vi "binarySearch.vi"(2 "Target":variant, 3 "Array":variant[](array[variant])) -> (0 "Itr to complete":i32, 1 "Result":i32)   [LabVIEW 2020]
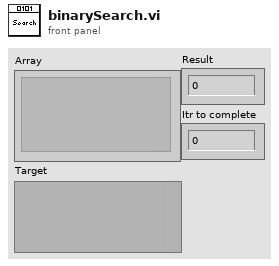
[diagram p1: front panel]
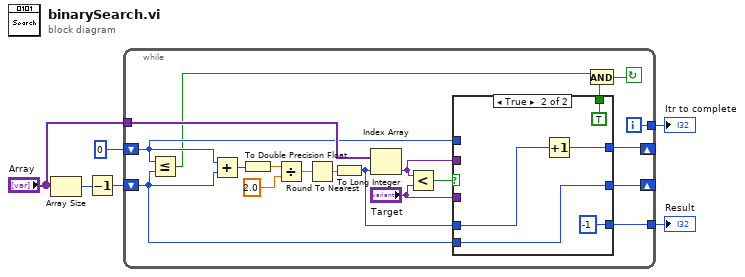
[diagram p0: block diagram]
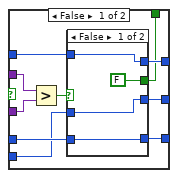
[diagram p2: hidden frame]
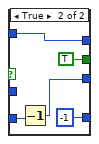
[diagram p3: hidden frame]
diagram:
  n1 = Array Size(array="Array") -> (size(s)=w6:i32)
  n2 = Decrement(x=w6) -> (x-1=w4:i32)
  n3 = while {
    tunnel: "Array" -> [w20]
    shift-right: [w18] -> _
    shift-left: 0 -> [w11]
    shift-right: [w14] -> _
    shift-left: w4 -> [w12]
    tunnel: [w13] -> w2
    tunnel: [w10] -> w1
    i -> [w10]
    stop <- w9 continue-if-true
    n4 = Less Or Equal?(x=w11, y=w12) -> (x <= y?=w8:bool)
    n5 = Add(x=w11, y=w12) -> (x+y=w25:i32)
    n6 = To Double Precision Float(number=w25) -> (double precision float=w24:dbl)
    n7 = Divide(x=w24, y=2.0) -> (x/y=w22:dbl)
    n8 = Round To Nearest(number=w22) -> (nearest integer value=w21:dbl)
    n9 = To Long Integer(number=w21) -> (32bit integer=w15:i32)
    n10 = Index Array(array=w20, index=w15) -> (element=w17:variant)
    n11 = Less?(x=w17, y="Target") -> (x < y?=w19:bool)
    n12 = case shown="True" w19 {
      tunnel: w15 -> [w32 w48]
      tunnel: [w28 w49] -> w18
      tunnel: w17 -> [w35 _]
      tunnel: "Target" -> [w34 _]
      tunnel: [w31 w47] -> w14
      tunnel: [w30 -1] -> w13
      tunnel: w12 -> [w27 w47]
      tunnel: w11 -> [w29 _]
      tunnel: [w26 TRUE] -> w7
      frame False {
        n13 = Greater?(x=w35, y=w34) -> (0:w33:bool)
        n14 = case shown="False" w33 {
          tunnel: w32 -> [w39 w44]
          tunnel: [w38 w43] -> w31
          tunnel: [w39 -1] -> w30
          tunnel: w29 -> [w37 w42]
          tunnel: [w37 w42] -> w28
          tunnel: w27 -> [w38 _]
          tunnel: [FALSE TRUE] -> w26
          frame False {
          }
          frame True {
            n15 = Decrement(x=w44) -> (x-1=w43:i32)
          }
        }
      }
      frame True {
        n16 = Increment(x=w48) -> (x+1=w49:i32)
      }
    }
    n17 = And(x=w8, y=w7) -> (x .and. y?=w9:bool)
  }
  "Result" <- w2
  "Itr to complete" <- w1
